vi "Test_ConstructTransport_InvalidPath_Error.vi"(8 "error in (no error)":errorcluster, 11 "TestCase in":refnum<class "TestPersistToDiskTransport.lvclass">) -> (0 "error out":errorcluster, 3 "TestCase out":refnum<class "TestPersistToDiskTransport.lvclass">)   [LabVIEW 2017, in "TestPersistToDiskTransport.lvclass"]
uses:
  TestPersistToDiskTransport.lvclass
  Source/Concrete/PersistToDiskTransport/PersistToDiskTransport.lvclass/PersistToDiskTransport.ctl
  <vilib>/Utility/error.llb/Clear Errors.vi
  Source/Concrete/PersistToDiskTransport/PersistToDiskTransport.lvclass
panel:
  out "Return Error":errorcluster
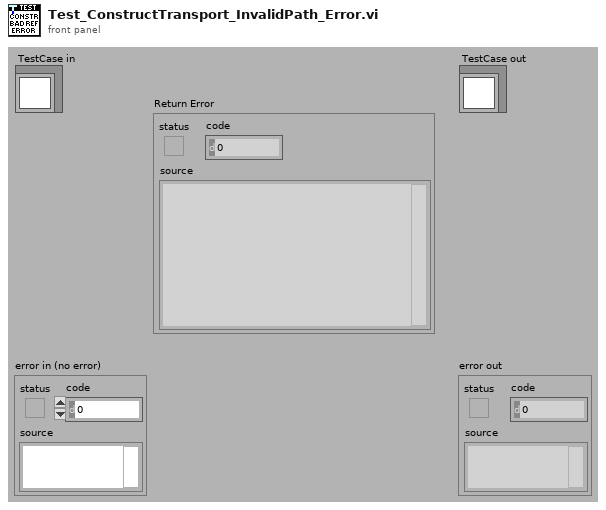
[diagram p1: front panel]
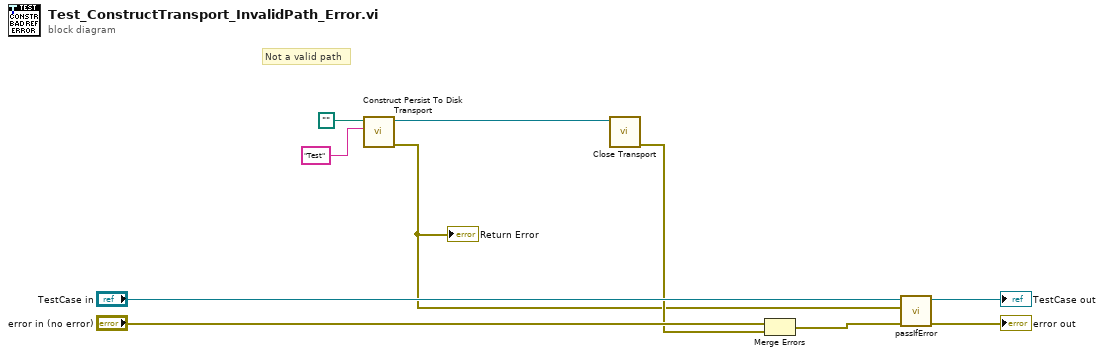
[diagram p0: block diagram]
diagram:
  # "Not a valid path"
  n1 = call "Construct Persist To Disk Transport.vi"("Datum Name"="Test" ("Key Name"), "Folder Path"=path "") -> ("error out"=w3:errorcluster, "PersistToDiskTransport"=w6:refnum<class "PersistToDiskTransport.lvclass">)  [unwired: 8 in]
  "Return Error" <- w3
  n2 = call-dynamic "Close Transport.vi"("ITransport in"=w6) -> ("error out"=w4:errorcluster)  [unwired: 10 in]
  n3 = Merge Errors("error in (no error)", w4) -> (w7:errorcluster)
  n4 = call-dynamic "passIfError.vi"("error in (no error)"=w7, "error"=w3, "TestCase in"="TestCase in") -> ("error out"=→"error out":errorcluster, "TestCase out"=→"TestCase out":refnum<class "TestPersistToDiskTransport.lvclass">)  [unwired: 7 in]
